vi "VHM-getSettings.vi"(8 "error in (no error)":errorcluster, 11 "VHM-VNA_Hardware_Manager in":refnum<class "VHM-VNA_Hardware_Manager.lvclass">) -> (0 "error out":errorcluster, 2 "Settings status":T1, 3 "VHM-VNA_Hardware_Manager out":refnum<class "VHM-VNA_Hardware_Manager.lvclass">)   [LabVIEW 2020, in "VHM-VNA_Hardware_Manager.lvlib" / "VHM-VNA_Hardware_Manager.lvclass"]
uses:
  VHM-VNA_Hardware_Manager.lvclass
  classes/vna-drivers/liteVNA/VD-settings_status.ctl
  VHM-VNA_Hardware_Manager.lvclass/VHM-VNA_Hardware_Manager.ctl
  classes/vna-drivers/liteVNA/VD-LV-LiteVNA.lvclass
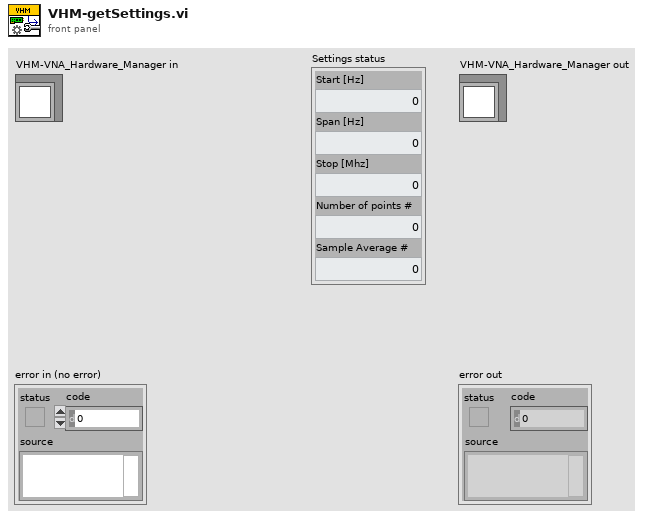
[diagram p1: front panel]
types:
  T1 = typedef "VD-LV-LiteVNA.lvclass/VD-settings_status.ctl" = cluster{"Start [Hz]":u64, "Span [Hz]":u64, "Stop [Mhz]":u64, "Number of points #":u16, "Sample Average #":u16}
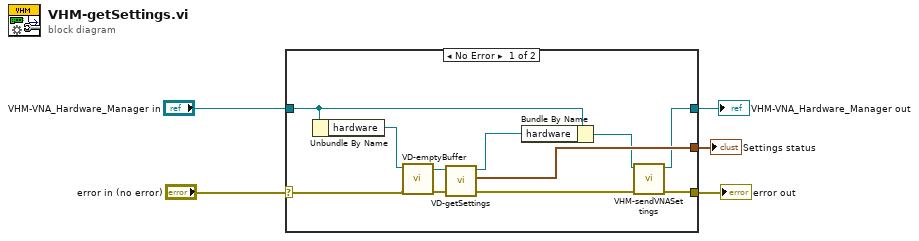
[diagram p0: block diagram]
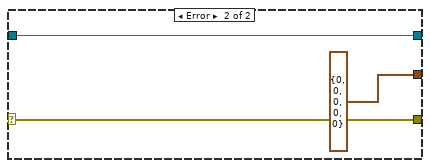
[diagram p2: hidden frame]
diagram:
  n1 = case shown="No Error" "error in (no error)" {
    selector: "error in (no error)" -> [w10 w19]
    tunnel: [w8 w19] -> w4
    tunnel: [w6 w18] -> w2
    tunnel: "VHM-VNA_Hardware_Manager in" -> [w16 w18]
    tunnel: [w14 T1 {"Start [Hz]"=0, "Span [Hz]"=0, "Stop [Mhz]"=0, "Number of points #"=0, "Sample Average #"=0} ("Settings status")] -> w1
    frame No Error {
      n2 = Unbundle By Name(w16) -> ("hardware"=w11:refnum<class "VD-LV-LiteVNA.lvclass">)
      n3 = call-dynamic "VD-emptyBuffer.vi"("error in (no error)"=w10, "VD-LV-LiteVNA in"=w11) -> ("error out"=w13:errorcluster, "VD-LV-LiteVNA out"=w12:refnum<class "VD-LV-LiteVNA.lvclass">)  [unwired: 5 in, 3 out]
      n4 = call "VD-getSettings.vi"("error in (no error)"=w13, "VD-LV-LiteVNA in"=w12) -> ("error out"=w9:errorcluster, "Settings status"=w14:T1, "VD-LV-LiteVNA out"=w15:refnum<class "VD-LV-LiteVNA.lvclass">)  [unwired: 7 in]
      n5 = Bundle By Name(cluster=w16, "hardware"=w15) -> (w7:refnum<class "VHM-VNA_Hardware_Manager.lvclass">)
      n6 = call "VHM-sendVNASettings.vi"("error in (no error)"=w9, "VHM-VNA_Hardware_Manager in"=w7) -> ("error out"=w8:errorcluster, "VHM-VNA_Hardware_Manager out"=w6:refnum<class "VHM-VNA_Hardware_Manager.lvclass">)  [unwired: 8 in]
    }
    frame Error {
    }
  }
  "error out" <- w4
  "VHM-VNA_Hardware_Manager out" <- w2
  "Settings status" <- w1
